vi "paths for z-scan.vi"(8 "Error in":errorcluster, 10 "file path":cluster{"File-name for z-scan":path}={"File-name for z-scan"=path "C:/Users/microscope/Desktop/Dropbox/RIP/Messungen/SM980_PTP_Errors_"}, 11 "Action":T1) -> (0 "Error out":errorcluster, 2 "file path out":cluster{"File-name for z-scan":path}={"File-name for z-scan"=path "C:/Users/microscope/Desktop/Dropbox/RIP/Messungen/SM980_PTP_Errors_"})   [LabVIEW 2011]
doc: "Functional Global Variable for the algorithm settings. The used method as well as the max. Iteration steps and the tolerance can be given. In addition, the algorithm can be told to use boundaries (if possible)."
uses:
  controls/FGV_Action.ctl
panel:
  # "Input"
  # "Output"
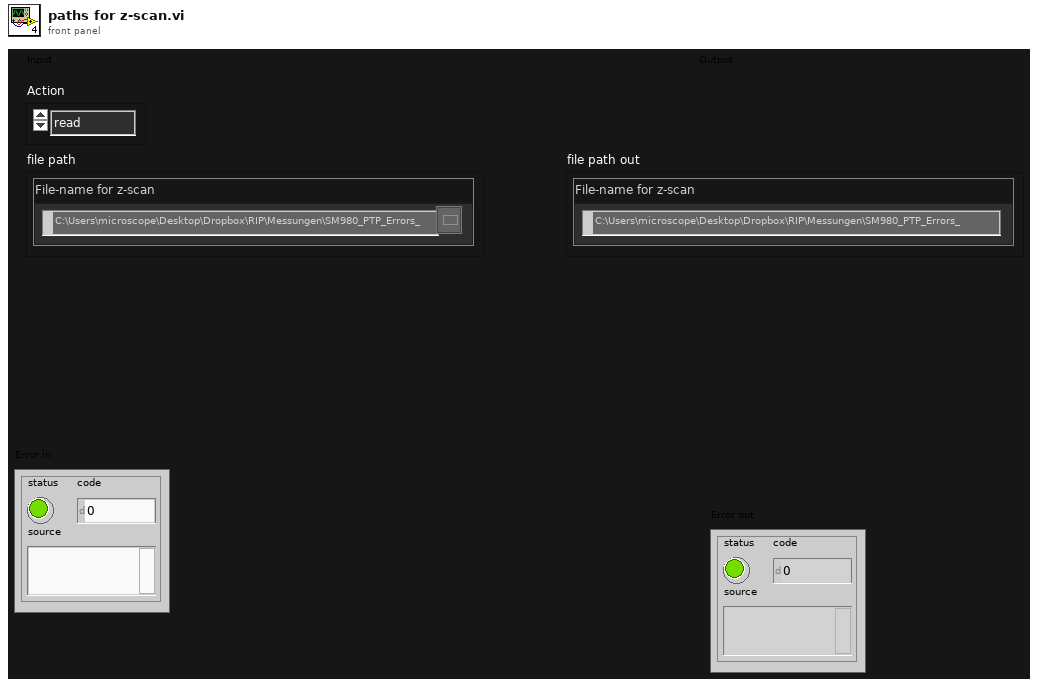
[diagram p1: front panel]
types:
  T1 = typedef "FGV_Action.ctl" = enum16{"read", "write"}
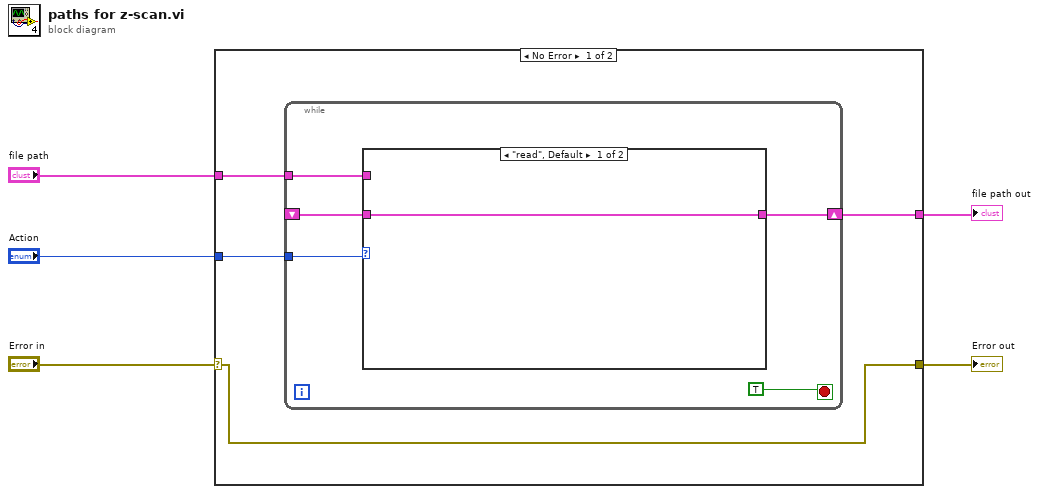
[diagram p0: block diagram]
diagram:
  n1 = case shown="No Error" "Error in" {
    selector: "Error in" -> [w6 w18]
    tunnel: "Action" -> [w9 _]
    tunnel: [w6 w18] -> w4
    tunnel: "file path" -> [w8 w17]
    tunnel: [w7 w17] -> w2
    frame No Error {
      n2 = while {
        tunnel: w9 -> [w13]
        tunnel: w8 -> [w12]
        shift-right: [w10] -> w7
        shift-left: _ -> [w11]
        stop <- TRUE stop-if-true
        n3 = case shown="\"read\", Default" w13 {
          tunnel: w12 -> [_ w16]
          tunnel: w11 -> [w15 _]
          tunnel: [w15 w16] -> w10
          frame "read", Default {
          }
          frame "write" {
          }
        }
      }
    }
    frame Error {
    }
  }
  "Error out" <- w4
  "file path out" <- w2
